vi "Make_odour_chemical_list_strings.vi"(11 "Odour component data":T1) -> (3 "Array":string[][](array[string]))   [LabVIEW 2016]
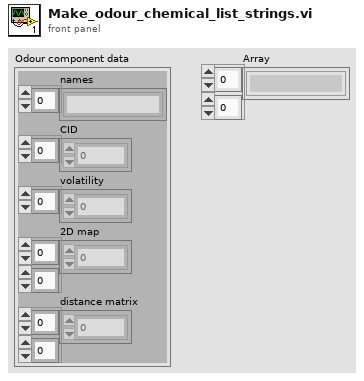
[diagram p1: front panel]
types:
  T1 = cluster{"names":string[], "CID":i32[], "volatility":dbl[], "2D map":dbl[][], "distance matrix":dbl[][]}
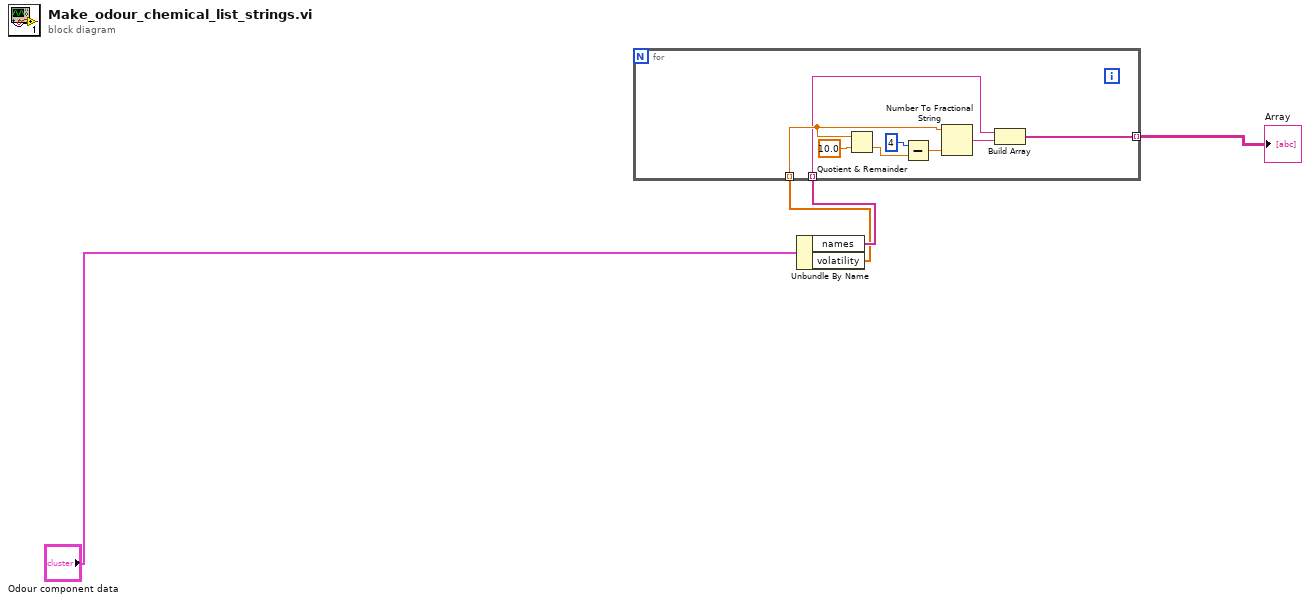
[diagram p0: block diagram]
diagram:
  n1 = Unbundle By Name("Odour component data") -> ("names"=w3:string[], "volatility"=w2:dbl[])
  n2 = for {
    tunnel: [w11] -> w1 mode=indexing
    tunnel: w2 -> [w6] mode=indexing
    tunnel: w3 -> [w5] mode=indexing
    n3 = Quotient & Remainder(x=w6, y=10.0) -> (floor(x/y)=w8:dbl)  [unwired: 1 out]
    n4 = Subtract(x=i16 4 ("precision (6)"), y=w8) -> (x-y=w7:dbl)
    n5 = Number To Fractional String(number=w6, precision (6)=w7) -> (F-format string=w12:string)  [unwired: 2 in]
    n6 = Build Array(w5, w12) -> (w11:string[])
  }
  "Array" <- w1
